vi "LabView360-6-布局.vi"() -> ()   [LabVIEW 2017]
panel:
  in  "布尔 5":bool
  in  "布尔 4":bool
  in  "布尔 3":bool
  in  "布尔 2":bool
  in  "布尔":bool
  in  "字符串 2":string
  in  "字符串":string
  out "波形图":dbl[](graph)
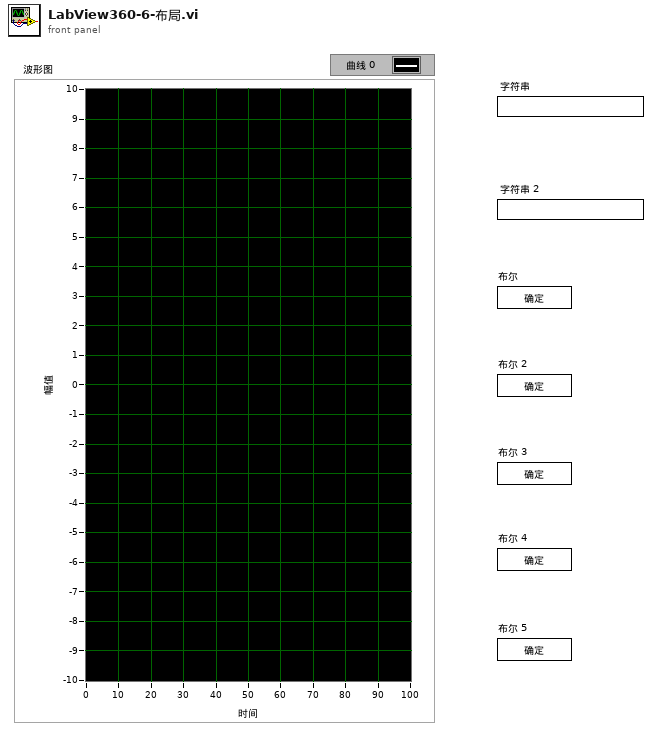
[diagram p1: front panel]
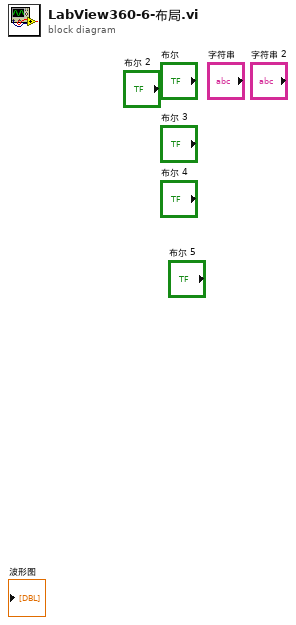
[diagram p0: block diagram]
diagram:
